vi "_052.vi"() -> ()   [LabVIEW 2024]
panel:
  out "appended array":string[](array[string])
  out "String 2":string
  in  "String":string
  # "Type Cast Function :"
  # "(using String & Hexa Decimal)"
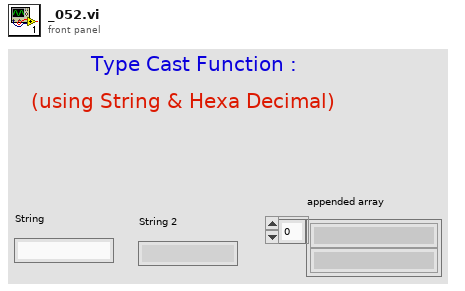
[diagram p1: front panel]
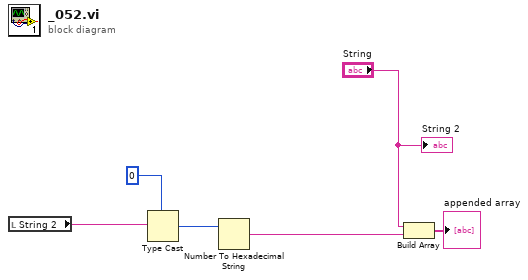
[diagram p0: block diagram]
diagram:
  n1 = local read "String 2"() -> (w4:string)
  n2 = Type Cast(type=i64 0, x=w4) -> (*(type *) &x=w2:i64)
  n3 = Number To Hexadecimal String(2:w2) -> (0:w1:string)  [unwired: 1 in]
  n4 = Build Array("String", w1) -> (→"appended array":string[])
  "String 2" <- "String"
